vi "Swerve Drive 6181.vi"(0 "X":dbl(slide) scale=-1.0..1.0, 1 "Y":dbl(slide) scale=1.0..-1.0, 2 "Z":dbl(knob) scale=1.0..-1.0, 3 "Robot-Centric":bool, 4 "Auto Controls":bool) -> ()   [LabVIEW 2020]
uses:
  <vilib>/Rock Robotics/Network Tables/NT Write Number.vi
panel:
  in  "Robot Length":dbl=33.0
  in  "Robot Width":dbl=25.0
  # "SWERVE DRIVE\nVersion 3.1\n\nCory Lynch\nApple Pi Robotics\nTeam 2067"
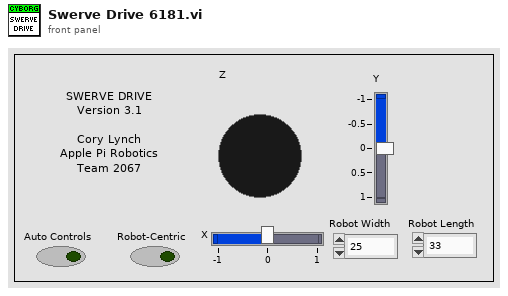
[diagram p1: front panel]
types:
  T1 = enum16{"Back Left", "Back Right", "Front Left", "Front Right"}
  T2 = cluster{"Yaw":dbl, "Roll":dbl, "Pitch":dbl, "Heading":dbl, "Fused Heading":dbl}
  T3 = typedef "WPI_MotorControlDeviceRef.ctl" = cluster{"DeviceStatus":errorcluster, "Type":T4, "PWM":cluster{"PWM Channel":T5, "DeadBand":T6}, "CAN":cluster{"Device Number":u8, "SetOutput VI Ref":variant, "GetOutput VI Ref":variant, "Enable VI Ref":variant, "Disable VI Ref":variant, "Data":variant}, "Invert":bool, "DIO PWM":cluster{"PWM \"Enable\" Channel":T5, "DIOChannel":T7, "PWM Rate":dbl}}
  T4 = typedef "WPI_MotorControlType.ctl" = enum16{"PWM", "CAN", "DIO PWM"}
  T5 = typedef "FPGA_DIOPWMChannel.ctl" = enum8{"PWM 0", "PWM 1", "PWM 2", "PWM 3", "PWM 4", "PWM 5", "PWM 6", "PWM 7", "PWM 8", "PWM 9", "PWM MXP 0", "PWM MXP 1", "PWM MXP 2", "PWM MXP 3", "PWM MXP 4", "PWM MXP 5", "PWM MXP 6", "PWM MXP 7", "PWM MXP 8", "PWM MXP 9", "Invalid"}
  T6 = typedef "WPI_PWMDeadband.ctl" = cluster{"Name":string, "maxPositivePwm":i32, "minPositivePwm":i32, "centerPwm":i32, "maxNegativePwm":i32, "minNegativePwm":i32, "angularRange":u16}
  T7 = typedef "FPGA_DIOChannel.ctl" = enum8{"DIO 0", "DIO 1", "DIO 2", "DIO 3", "DIO 4", "DIO 5", "DIO 6", "DIO 7", "DIO 8", "DIO 9", "DIO MXP 0", "DIO MXP 1", "DIO MXP 2", "DIO MXP 3", "DIO MXP 4", "DIO MXP 5", "DIO MXP 6", "DIO MXP 7", "DIO MXP 8", "DIO MXP 9", "DIO MXP 10", "DIO MXP 11", "DIO MXP 12", "DIO MXP 13", "DIO MXP 14", "DIO MXP 15", "SPI Port CS1", "SPI Port CS2", "SPI Port CS3", "SPI Port MISO", "SPI Port MOSI", "Invalid"}
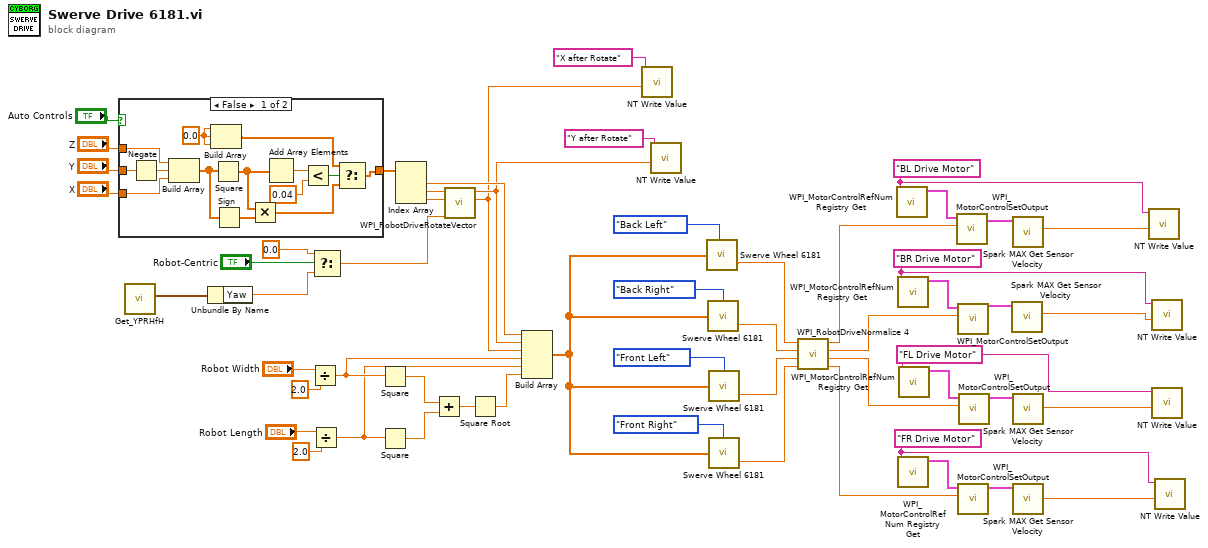
[diagram p0: block diagram]
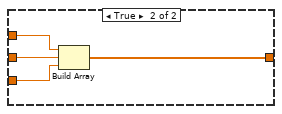
[diagram p2: hidden frame]
diagram:
  w11 = "FR Drive Motor" ("refnum name")
  w13 = "FL Drive Motor" ("refnum name")
  w14 = "BR Drive Motor" ("refnum name")
  w16 = "BL Drive Motor" ("refnum name")
  n1 = case shown="False" "Auto Controls" {
    tunnel: "Y" -> [w67 w73]
    tunnel: "X" -> [w61 w74]
    tunnel: "Z" -> [w57 w71]
    tunnel: [w58 w72] -> w36
    frame False {
      w65 = 0.0 ("element")
      n2 = Negate(x=w67) -> (-x=w60:dbl)
      n3 = Build Array(w57, w60, w61) -> (w64:dbl[])
      n4 = Build Array(w65, w65, w65) -> (w66:dbl[])
      n5 = Square(x=w64) -> (x^2=w62:dbl[])
      n6 = Sign(1:w64) -> (0:w63:dbl[])
      n7 = Multiply(x=w62, y=w63) -> (x*y=w59:dbl[])
      n8 = Add Array Elements(numeric array=w62) -> (sum=w70:dbl)
      n9 = Less?(x=w70, y=0.04 ("x")) -> (x < y?=w68:bool)
      n10 = Select(t=w66, s=w68, f=w59) -> (s? t:f=w58:dbl[])
    }
    frame True {
      n11 = Build Array(w71, w73, w74) -> (w72:dbl[])
    }
  }
  n12 = call <vilib>:"Get_YPRHfH.vi"() -> ("YRPHfH"=w5:T2)  [unwired: 11 in]
  n13 = Unbundle By Name(w5) -> ("Yaw"=w31:dbl)
  n14 = Divide(x="Robot Width", y=2.0) -> (x/y=w30:dbl)
  n15 = Divide(x="Robot Length", y=2.0) -> (x/y=w29:dbl)
  n16 = Select(t=0.0, s="Robot-Centric", f=w31) -> (s? t:f=w35:dbl)
  n17 = Square(x=w30) -> (x^2=w46:dbl)
  n18 = Square(x=w29) -> (x^2=w47:dbl)
  n19 = Index Array(array=w36) -> (element #1=w34:dbl, element #2=w37:dbl, element #3=w40:dbl)  [unwired: 3 in]
  n20 = Add(x=w46, y=w47) -> (x+y=w45:dbl)
  n21 = call <vilib>:"WPI_RobotDriveRotateVector.vi"("Angle"=w35, "X"=w40, "Y"=w37) -> ("X'"=w2:dbl, "Y'"=w4:dbl)  [unwired: 7 out]
  n22 = Square Root(x=w45) -> (sqrt(x)=w28:dbl)
  n23 = Build Array(w34, w4, w2, w30, w29, w28) -> (w22:dbl[])
  n24 = call-poly <vilib>:"NT Write Value.vi"("value"=w2, "name"="X after Rotate" ("Name")) -> ()  [unwired: 9 in, 1 out]
  n25 = call-poly <vilib>:"NT Write Value.vi"("value"=w4, "name"="Y after Rotate" ("Name")) -> ()  [unwired: 9 in, 1 out]
  n26 = call "Swerve Wheel 6181.vi"("Wheel"=T1."Back Left", "Inputs"=w22) -> ("Speed"=w27:dbl)  [unwired: 3 in]
  n27 = call "Swerve Wheel 6181.vi"("Wheel"=T1."Back Right", "Inputs"=w22) -> ("Speed"=w25:dbl)  [unwired: 3 in]
  n28 = call "Swerve Wheel 6181.vi"("Wheel"=T1."Front Left", "Inputs"=w22) -> ("Speed"=w24:dbl)  [unwired: 3 in]
  n29 = call "Swerve Wheel 6181.vi"("Wheel"=T1."Front Right", "Inputs"=w22) -> ("Speed"=w23:dbl)  [unwired: 3 in]
  n30 = call <vilib>:"WPI_RobotDriveNormalize 4.vi"("D"=w23, "C"=w24, "B"=w25, "A"=w27) -> ("D'"=w49:dbl, "C'"=w50:dbl, "B'"=w51:dbl, "A'"=w52:dbl)
  n31 = call <vilib>:"WPI_MotorControlRefNum Registry Get.vi"("refnum name"=w16) -> ("MotorControlDevRef"=w56:T3)  [unwired: 9 in, 1 out]
  n32 = call <vilib>:"WPI_MotorControlRefNum Registry Get.vi"("refnum name"=w14) -> ("MotorControlDevRef"=w55:T3)  [unwired: 9 in, 1 out]
  n33 = call <vilib>:"WPI_MotorControlRefNum Registry Get.vi"("refnum name"=w11) -> ("MotorControlDevRef"=w53:T3)  [unwired: 9 in, 1 out]
  n34 = call <vilib>:"WPI_MotorControlRefNum Registry Get.vi"("refnum name"=w13) -> ("MotorControlDevRef"=w54:T3)  [unwired: 9 in, 1 out]
  n35 = call <vilib>:"WPI_MotorControlSetOutput.vi"("Output"=w52, "MotorControlDevRef"=w56) -> ("MotorControlDevRef"=w21:T3)  [unwired: 7 in, 2 out]
  n36 = call <vilib>:"WPI_MotorControlSetOutput.vi"("Output"=w51, "MotorControlDevRef"=w55) -> ("MotorControlDevRef"=w20:T3)  [unwired: 7 in, 2 out]
  n37 = call <vilib>:"WPI_MotorControlSetOutput.vi"("Output"=w49, "MotorControlDevRef"=w53) -> ("MotorControlDevRef"=w18:T3)  [unwired: 7 in, 2 out]
  n38 = call <vilib>:"WPI_MotorControlSetOutput.vi"("Output"=w50, "MotorControlDevRef"=w54) -> ("MotorControlDevRef"=w19:T3)  [unwired: 7 in, 2 out]
  n39 = call <vilib>:"Spark MAX Get Sensor Velocity.vi"("MotorControlDevRef in"=w20) -> ("Sensor Velocity"=w15:dbl)  [unwired: 7 in, 3 out]
  n40 = call <vilib>:"Spark MAX Get Sensor Velocity.vi"("MotorControlDevRef in"=w21) -> ("Sensor Velocity"=w17:dbl)  [unwired: 7 in, 3 out]
  n41 = call <vilib>:"Spark MAX Get Sensor Velocity.vi"("MotorControlDevRef in"=w19) -> ("Sensor Velocity"=w12:dbl)  [unwired: 7 in, 3 out]
  n42 = call <vilib>:"Spark MAX Get Sensor Velocity.vi"("MotorControlDevRef in"=w18) -> ("Sensor Velocity"=w10:dbl)  [unwired: 7 in, 3 out]
  n43 = call-poly <vilib>:"NT Write Value.vi"("value"=w17, "name"=w16) -> ()  [unwired: 9 in, 1 out]
  n44 = call-poly <vilib>:"NT Write Value.vi"("value"=w15, "name"=w14) -> ()  [unwired: 9 in, 1 out]
  n45 = call-poly <vilib>:"NT Write Value.vi"("value"=w12, "name"=w13) -> ()  [unwired: 9 in, 1 out]
  n46 = call-poly <vilib>:"NT Write Value.vi"("value"=w10, "name"=w11) -> ()  [unwired: 9 in, 1 out]
